vi "isRefValid.vi"(8 "error in (no error)":errorcluster, 11 "xwpfHeader in":refnum<class "xwpfHeader_Footer.lvclass">) -> (0 "error out":errorcluster, 3 "xwpfHeader out":refnum<class "xwpfHeader_Footer.lvclass">)   [LabVIEW 2017, in "Word_Specific.lvlib" / "xwpfHeader_Footer.lvclass"]
uses:
  xwpfHeader_Footer.lvclass
  xwpfHeader_Footer.lvclass/xwpfHeader_Footer.ctl
  <vilib>/Utility/error.llb/Error Cluster From Error Code.vi
  <vilib>/ErrorRing/Error Ring.xnode
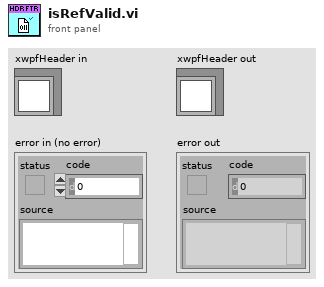
[diagram p1: front panel]
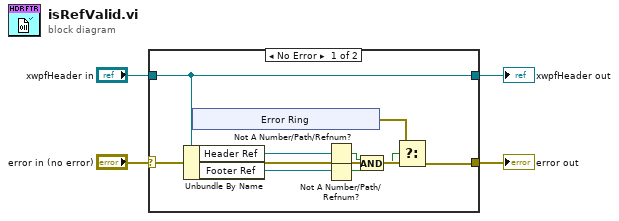
[diagram p0: block diagram]
diagram:
  n1 = case shown="No Error" "error in (no error)" {
    selector: "error in (no error)" -> [w11 w20]
    tunnel: [w10 w20] -> w1
    tunnel: [w13 w19] -> w3
    tunnel: "xwpfHeader in" -> [w13 w19]
    frame No Error {
      n2 = Unbundle By Name(w13) -> ("Header Ref"=w9:refnum<k24>, "Footer Ref"=w8:refnum<k24>)
      n3 = xnode "Error Ring"() -> ("error out"=w12:errorcluster)
      n4 = Not A Number/Path/Refnum?(number/path/refnum=w9) -> (NaN/Path/Refnum?=w6:bool)
      n5 = Not A Number/Path/Refnum?(number/path/refnum=w8) -> (NaN/Path/Refnum?=w7:bool)
      n6 = And(x=w6, y=w7) -> (x .and. y?=w5:bool)
      n7 = Select(t=w12, s=w5, f=w11) -> (s? t:f=w10:errorcluster)
    }
    frame Error {
    }
  }
  "error out" <- w1
  "xwpfHeader out" <- w3
